vi "冒泡排序.vi"() -> ()   [LabVIEW 2016]
panel:
  in  "等待时间（毫秒）":u32=10
  out "无交换":bool
  out "交换次数":dbl
  out "循环次数":dbl
  out "排序前":i16[](array[numeric])
  out "排序后":i16[](array[numeric])
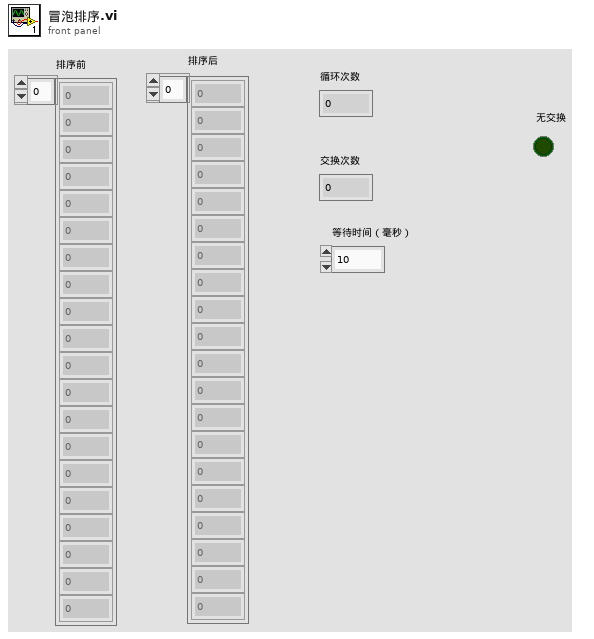
[diagram p1: front panel]
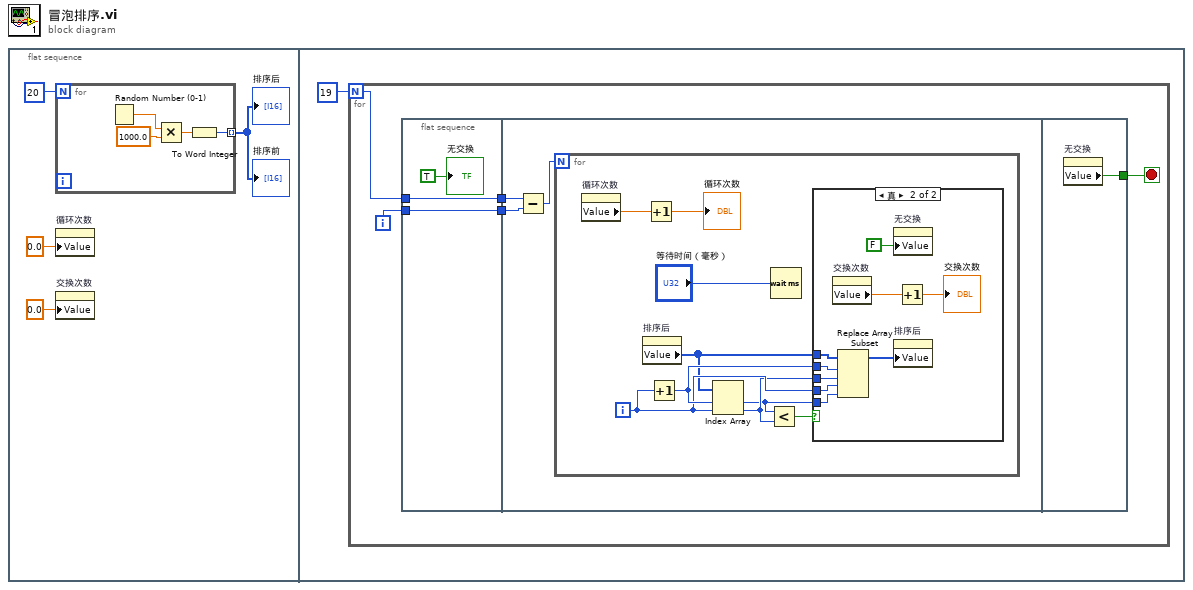
[diagram p0: block diagram]
diagram:
  n1 = flat-sequence {
    frame #0 {
      n2 = for {
        N: 20 -> [_]
        tunnel: [w5] -> w4 mode=indexing
        n3 = Random Number (0-1)() -> (number: 0 to 1=w8:dbl)
        n4 = Multiply(x=w8, y=1000.0) -> (x*y=w6:dbl)
        n5 = To Word Integer(number=w6) -> (16bit integer=w5:i16)
      }
      "排序后" <- w4
      "排序前" <- w4
      n6 = property on="循环次数" class="DigNum (严格)"("Value"=0.0 ("循环次数")) -> ()  [unwired: 2 in, 2 out]
      n7 = property on="交换次数" class="DigNum (严格)"("Value"=0.0 ("交换次数")) -> ()  [unwired: 2 in, 2 out]
    }
    frame #1 {
      n8 = for {
        N: 19 -> [w14]
        i -> [w13]
        stop <- w10 stop-if-true
        n9 = flat-sequence {
          tunnel: w13 -> [w16]
          tunnel: w14 -> [w17]
          tunnel: [w17] -> w12
          tunnel: [w16] -> w11
          tunnel: w12 -> [w19]
          tunnel: w11 -> [w18]
          tunnel: [w39] -> w10
          frame #0 {
            "无交换" <- TRUE ("无交换")
          }
          frame #1 {
            n10 = Subtract(x=w19, y=w18) -> (x-y=w20:i32)
            n11 = for {
              N: w20 -> [_]
              i -> [w27]
              n12 = property on="循环次数" class="DigNum (严格)"() -> ("Value"=w22:dbl)  [unwired: 2 in, 2 out]
              n13 = property on="排序后" class="Arr (严格)"() -> ("Value"=w24:i16[])  [unwired: 2 in, 2 out]
              n14 = Increment(x=w22) -> (x+1=→"循环次数":dbl)
              n15 = Increment(x=w27) -> (x+1=w28:i32)
              n16 = Index Array(array=w24, index #1=w28, index #2=w27) -> (element #1=w25:i16, element #2=w26:i16)
              n17 = Less?(x=w25, y=w26) -> (x < y?=w29:bool)
              n18 = Wait (ms)(milliseconds to wait="等待时间（毫秒）") -> ()  [unwired: 1 out]
              n19 = case shown="真" w29 {
                tunnel: w28 -> [_ w37]
                tunnel: w27 -> [_ w36]
                tunnel: w26 -> [_ w34]
                tunnel: w25 -> [_ w35]
                tunnel: w24 -> [_ w33]
                frame False {
                }
                frame True {
                  n20 = property on="交换次数" class="DigNum (严格)"() -> ("Value"=w31:dbl)  [unwired: 2 in, 2 out]
                  n21 = Replace Array Subset(array=w33, new element #1=w34, index #1=w37, new element #2=w35, index #2=w36) -> (w38:i16[])
                  n22 = property on="无交换" class="Bool (严格)"("Value"=FALSE ("无交换")) -> ()  [unwired: 2 in, 2 out]
                  n23 = property on="排序后" class="Arr (严格)"("Value"=w38) -> ()  [unwired: 2 in, 2 out]
                  n24 = Increment(x=w31) -> (x+1=→"交换次数":dbl)
                }
              }
            }
          }
          frame #2 {
            n25 = property on="无交换" class="Bool (严格)"() -> ("Value"=w39:bool)  [unwired: 2 in, 2 out]
          }
        }
      }
    }
  }
